vi "PH_gentec_M-Link.set Trigger Level.vi"(0 "i ref in":refnum<vi>, 2 "VISA resource in":refnum<visa-resource-name>, 5 "error in":errorcluster) -> (11 "Timeout":bool, 13 "Data read":string[](array[string]), 14 "i ref out":refnum<vi>, 16 "VISA resource out":refnum<visa-resource-name>, 17 "Error":bool, 18 "Failure":bool, 19 "error out":errorcluster)   [LabVIEW 2014, in "PH_gentec_M-Link.lvlib"]
doc: "This VI writes wanted Settings to the Device and checks the result."
uses:
  PH_gentec_M-Link.lvlib
  instr.lib/Gentec-M-Link/gentec-M-Link - Driver.lvlib
  PH_Basics/PH_Powermeter_BaseClass/PH_Powermeter_BaseClass.lvlib
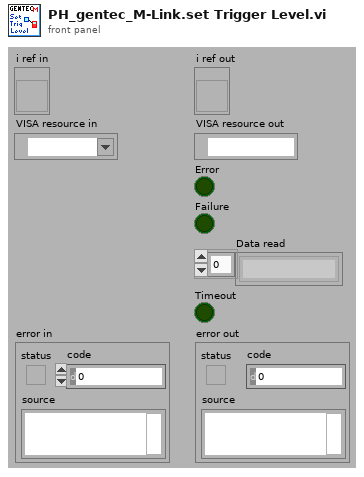
[diagram p1: front panel]
types:
  T1 = typedef "PH_Powermeter_BaseClass.lvlib/PH_Powermeter_BaseClass.i attribute.ctl" = cluster{"GUI References":T2, "Connection":T3, "Head Attributes":T5, "VISA resource":refnum<visa-resource-name>, "Energy":T6, "Service ID Energy":i32, "Wanted Settings":T7, "Current Settings":T7}
  T2 = typedef "PH_Powermeter_BaseClass.lvlib/PH_Powermeter_BaseClass.GUI Refs.ctl" = cluster{"Head Attributes":refnum<vi>, "Energy":refnum<vi>, "Connection":refnum<vi>, "VISA Resource":refnum<vi>, "Energy evolution":refnum<vi>, "Scaling Factor":refnum<vi>, "Range":refnum<vi>, "Wavelength":refnum<vi>, "Trigger Level":refnum<vi>, "Wanted Settings":refnum<vi>, "Current Settings":refnum<vi>}
  T3 = typedef "PH_Powermeter_BaseClass.lvlib/PH_Powermeter_BaseClass.Connection.ctl" = cluster{"failed checks":i8, "Timeout":bool, "Data read":string, "Failure":bool, "Error":bool, "State":T4}
  T4 = typedef "PH_Powermeter_BaseClass.lvlib/PH_Powermeter_BaseClass.State.ctl" = enum32{"off", "operating", "opened", "checked", "connected", "Sets to change", "running"}
  T5 = typedef "PH_Powermeter_BaseClass.lvlib/PH_Powermeter_BaseClass.Head Attributes.ctl" = cluster{"Instrument Type":string, "Head Version":string, "Head Name":string, "Serial Number":string, "Firmware":string, "Sensor Type":string, "MinimumRange":u32, "Maximum Range":u32, "Min Wavelength":i32, "Max Wavelength":i32}
  T6 = typedef "PH_Powermeter_BaseClass.lvlib/PH_Powermeter_BaseClass.Energy.ctl" = cluster{"current Value":dbl, "unscaled":dbl, "Scaling Factor":dbl}
  T7 = typedef "PH_Powermeter_BaseClass.lvlib/PH_gentec_BaseClass.Head Settings.ctl" = cluster{"Trigger Level":dbl, "Wavelength":u32, "Range":u32}
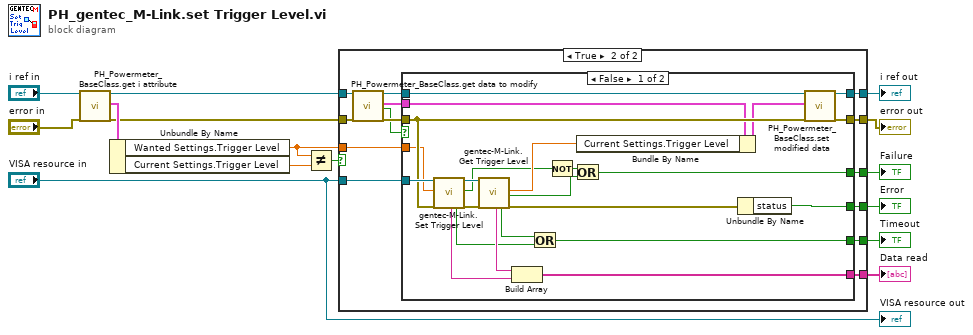
[diagram p0: block diagram]
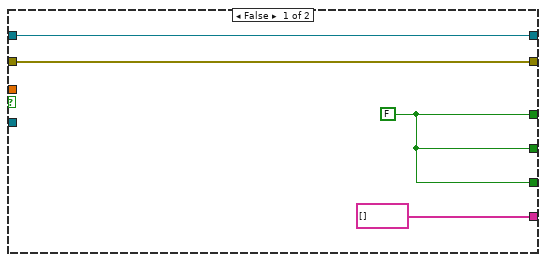
[diagram p2: hidden frame]
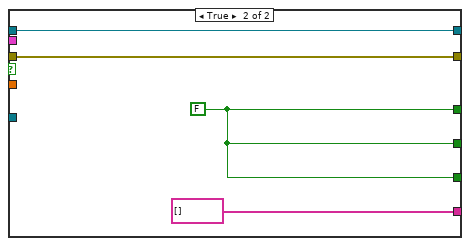
[diagram p3: hidden frame]
diagram:
  n1 = call "PH_Powermeter_BaseClass.get i attribute.vi"("i ref in"="i ref in", "error in (no error)"="error in") -> ("i ref out"=w8:refnum<vi>, "i attribute"=w11:T1, "error out"=w10:errorcluster)  [unwired: 15 in]
  n2 = Unbundle By Name(w11) -> ("Wanted Settings.Trigger Level"=w13:dbl, "Current Settings.Trigger Level"=w12:dbl)
  n3 = Not Equal?(x=w13, y=w12) -> (x != y?=w1:bool)
  n4 = case shown="True" w1 {
    tunnel: [w16 w33] -> w15
    tunnel: [w17 w32] -> w14
    tunnel: w13 -> [_ w31]
    tunnel: w10 -> [w16 w26]
    tunnel: w8 -> [w17 w25]
    tunnel: "VISA resource in" -> [_ w24]
    tunnel: [w19 w23] -> w5
    tunnel: [w19 w22] -> w4
    tunnel: [w19 w21] -> w3
    tunnel: [string[] [] w20] -> w2
    frame False {
      w19 = FALSE
    }
    frame True {
      n5 = call "PH_Powermeter_BaseClass.get data to modify.vi"("i ref in"=w25, "error in (no error)"=w26) -> ("i ref out"=w29:refnum<vi>, "i attribute"=w28:T1, "timed out"=w27:bool, "error out"=w30:errorcluster)  [unwired: 14 in]
      n6 = case shown="False" w27 {
        tunnel: w24 -> [w55 _]
        tunnel: [w51 w60] -> w32
        tunnel: [w50 w59] -> w33
        tunnel: w30 -> [w54 w59]
        tunnel: w29 -> [w56 w60]
        tunnel: w28 -> [w53 _]
        tunnel: w31 -> [w52 _]
        tunnel: [w48 w58] -> w23
        tunnel: [w47 w58] -> w22
        tunnel: [w46 w58] -> w21
        tunnel: [w45 string[] []] -> w20
        frame False {
          n7 = call "gentec-M-Link.Set Trigger Level.vi"("VISA resource In"=w55, "Trigger Level [%]"=w52, "error in (no error)"=w54) -> ("Data Read"=w40:string, "Read Timeout"=w37:bool, "VISA resource Out"=w44:refnum<visa-resource-name>, "Success"=w35:bool, "error out"=w43:errorcluster)  [unwired: 12 in]
          n8 = call "gentec-M-Link.Get Trigger Level.vi"("VISA resource In"=w44, "error in (no error)"=w43) -> ("Data Read"=w39:string, "Read Timeout"=w38:bool, "Trigger Level [%]"=w41:dbl, "Error"=w36:bool, "error out"=w42:errorcluster)  [unwired: 12 in, 1 out]
          n9 = Build Array(w39, w40) -> (w45:string[])
          n10 = Or(x=w38, y=w37) -> (x .or. y?=w46:bool)
          n11 = Not(x=w35) -> (.not. x?=w34:bool)
          n12 = Or(x=w34, y=w36) -> (x .or. y?=w47:bool)
          n13 = Bundle By Name(cluster=w53, "Current Settings.Trigger Level"=w41) -> (w49:T1)
          n14 = Unbundle By Name(w42) -> ("status"=w48:bool)
          n15 = call "PH_Powermeter_BaseClass.set modified data.vi"("i ref in"=w56, "i attribute"=w49, "error in (no error)"=w54) -> ("i ref out"=w51:refnum<vi>, "error out"=w50:errorcluster)  [unwired: 15 in]
        }
        frame True {
          w58 = FALSE
        }
      }
    }
  }
  "error out" <- w15
  "i ref out" <- w14
  "Error" <- w5
  "Failure" <- w4
  "Timeout" <- w3
  "Data read" <- w2
  "VISA resource out" <- "VISA resource in"
